vi "CSM Data Type.vi"() -> ()   [LabVIEW 2017]
uses:
  <vilib>/Utility/Data Type/Type Definitions/Data Type.ctl
  user.lib/_NEVSTOP/Communicable State Machine(CSM)/Utility/_support/CSM Data Type String to Enum(String).vi
  user.lib/_NEVSTOP/Communicable State Machine(CSM)/Communicable State Machine.lvlib
  <vilib>/Utility/Data Type/NI_Data Type.lvlib
panel:
  out "Array Dim 12":i32
  out "Secondary Type String 12":string
  out "Primary Type 12":T1
  out "Data Type String 12":string
  out "Array Dim 11":i32
  out "Secondary Type String 11":string
  out "Primary Type 11":T1
  out "Data Type String 11":string
  out "Array Dim 10":i32
  out "Secondary Type String 10":string
  out "Primary Type 10":T1
  out "Data Type String 10":string
  out "Array Dim 9":i32
  out "Secondary Type String 9":string
  out "Primary Type 9":T1
  out "Data Type String 9":string
  out "Array Dim 8":i32
  out "Secondary Type String 8":string
  out "Primary Type 8":T1
  out "Data Type String 8":string
  out "Array Dim 7":i32
  out "Secondary Type String 7":string
  out "Primary Type 7":T1
  out "Data Type String 7":string
  out "Array Dim 6":i32
  out "Secondary Type String 6":string
  out "Primary Type 6":T1
  out "Data Type String 6":string
  out "Array Dim 5":i32
  out "Secondary Type String 5":string
  out "Primary Type 5":T1
  out "Data Type String 5":string
  out "Array Dim 4":i32
  out "Secondary Type String 4":string
  out "Primary Type 4":T1
  out "Data Type String 4":string
  out "Array Dim 3":i32
  out "Secondary Type String 3":string
  out "Primary Type 3":T1
  out "Data Type String 3":string
  out "Array Dim 2":i32
  out "Secondary Type String 2":string
  out "Primary Type 2":T1
  out "Data Type String 2":string
  out "Data Type String":string
  out "Primary Type":T1
  out "Secondary Type String":string
  out "Array Dim":i32
  in  "Data 12":dbl[][](array[numeric])=[[3.12, 4.113, 2.3, 5.0, 5.0, 2.3, 4.11, 5.0]]
  in  "Data 11":T2(array[cluster])=[{"Name"="", "Child"={"Name"="ddd"}, "Bool"=FALSE}, {"Name"="ddd", "Child"={"Name"=""}, "Bool"=TRUE}]
  in  "Data 2":path=path "C:/ni-rt/data/a/2023.07.25"
  in  "Data 10":T3={"Name"="abc", "Child"={"Name"="ddd"}, "Bool"=FALSE}
  in  "Data 9":dbl[](array[numeric])=[3.12, 4.11, 5.0]
  in  "Data 8":enum16{"1 - aaaa", "2 - bbbb", "555 - ccccc"}(ring)=enum."555 - ccccc"
  in  "Data 7":enum16{"1 - aaaa", "2 - bbbb", "555 - ccccc"}(ring)=enum."555 - ccccc"
  in  "Data 6":enum16{"aaaa", "bbbb", "ccccc"}(ring)=enum."bbbb"
  in  "Data 5":dbl=3.1415926
  in  "Data 4":i32=66
  in  "Data 3":bool=TRUE
  in  "Data 1":string="abcd"
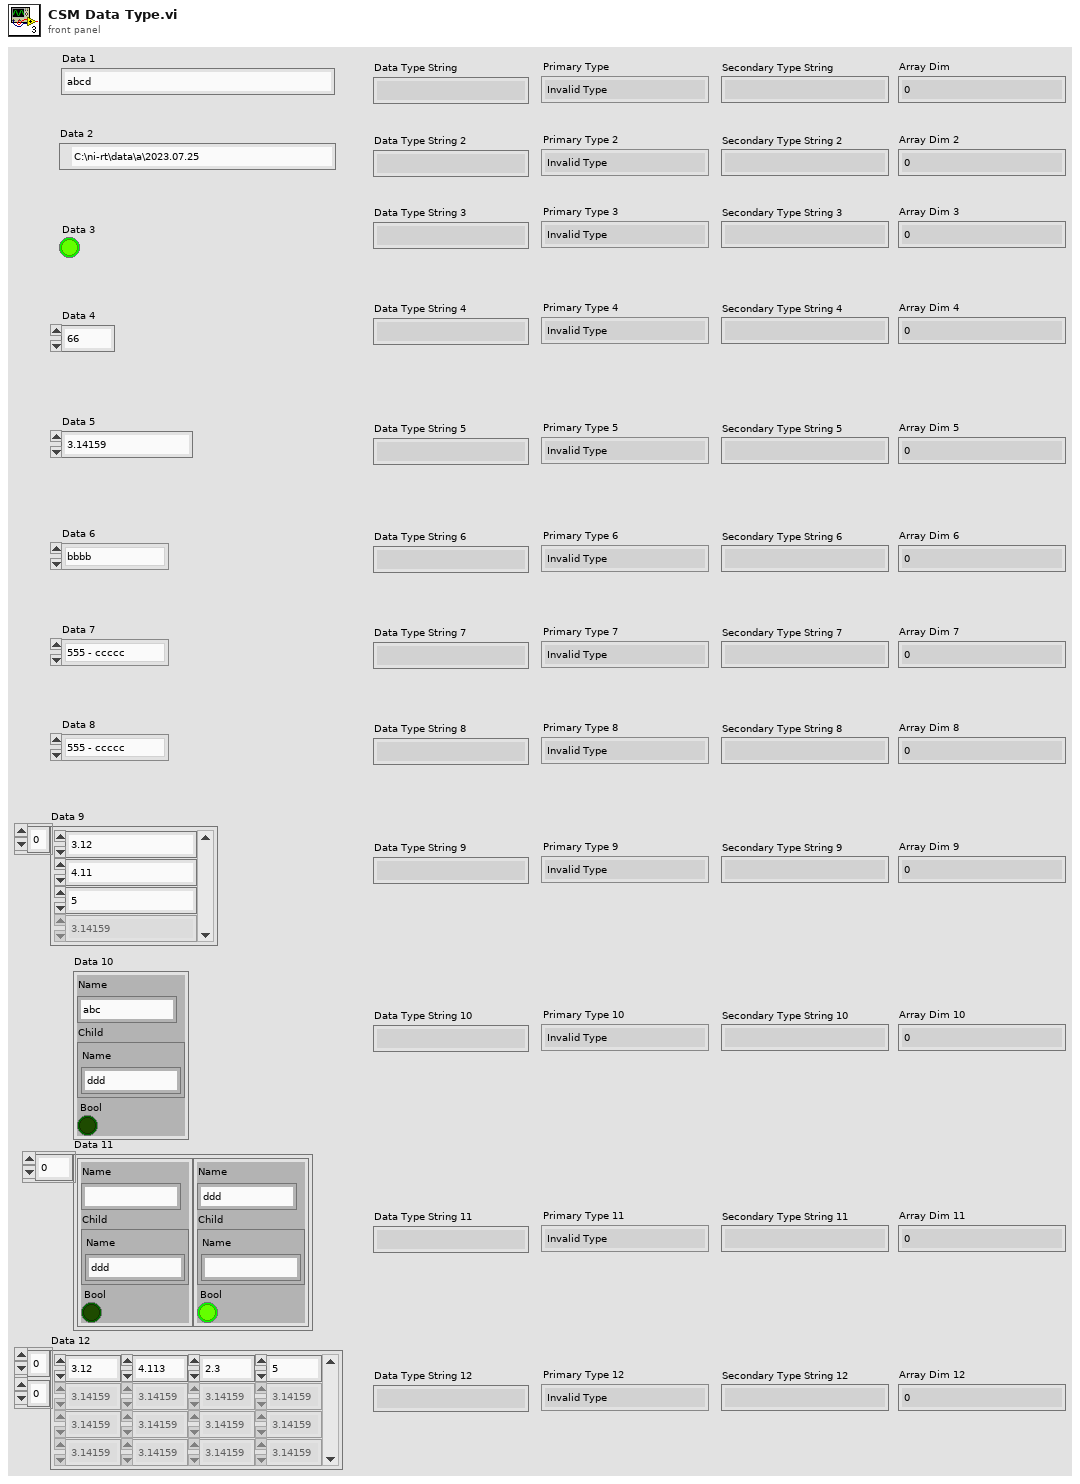
[diagram p1: front panel]
types:
  T1 = typedef "NI_Data Type.lvlib/Data Type.ctl" = enum8{"Invalid Type", "Void", "I8", "I16", "I32", "I64", "U8", "U16", "U32", "U64", "Single Float", "Double Float", "Extended Float", "Single Complex", "Double Complex", "Extended Complex", "Enum U8", "Enum U16", "Enum U32", "Enum U64", "Single Float With Unit", "Double Float With Unit", "Extended Float With Unit", "Single Complex with Unit", "Double Complex with Unit", "Extended Complex with Unit", "Boolean", "String", "Path", "Picture", "Tag", "Array", "Cluster", "Variant", "LV Variant", "Waveform", "Timestamp", "Digital Waveform", "Digital Data", "ExpressData", "Refnum", "External Data", "VI", "Poly VI", "LabVIEW Class Instance", "Fixed Point"}
  T2 = cluster{"Name":string, "Child":cluster{"Name":string}, "Bool":bool}[]
  T3 = cluster{"Name":string, "Child":cluster{"Name":string}, "Bool":bool}
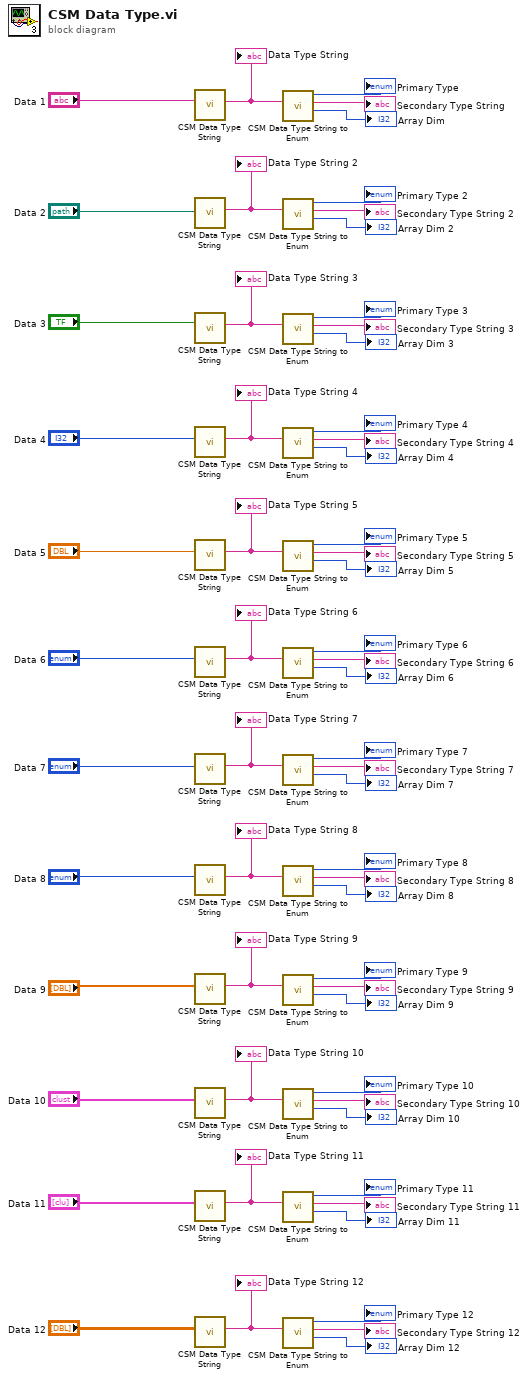
[diagram p0: block diagram]
diagram:
  n1 = call "CSM Data Type String.vi"("Data"="Data 1") -> ("Data Type String"=w60:string)  [unwired: 10 in]
  "Data Type String" <- w60
  n2 = call "CSM Data Type String.vi"("Data"="Data 2") -> ("Data Type String"=w52:string)  [unwired: 10 in]
  "Data Type String 2" <- w52
  n3 = call "CSM Data Type String.vi"("Data"="Data 3") -> ("Data Type String"=w50:string)  [unwired: 10 in]
  "Data Type String 3" <- w50
  n4 = call "CSM Data Type String.vi"("Data"="Data 4") -> ("Data Type String"=w42:string)  [unwired: 10 in]
  "Data Type String 4" <- w42
  n5 = call "CSM Data Type String.vi"("Data"="Data 5") -> ("Data Type String"=w40:string)  [unwired: 10 in]
  "Data Type String 5" <- w40
  n6 = call "CSM Data Type String.vi"("Data"="Data 6") -> ("Data Type String"=w32:string)  [unwired: 10 in]
  "Data Type String 6" <- w32
  n7 = call "CSM Data Type String.vi"("Data"="Data 7") -> ("Data Type String"=w30:string)  [unwired: 10 in]
  "Data Type String 7" <- w30
  n8 = call "CSM Data Type String.vi"("Data"="Data 8") -> ("Data Type String"=w22:string)  [unwired: 10 in]
  "Data Type String 8" <- w22
  n9 = call "CSM Data Type String.vi"("Data"="Data 9") -> ("Data Type String"=w20:string)  [unwired: 10 in]
  "Data Type String 9" <- w20
  n10 = call "CSM Data Type String.vi"("Data"="Data 10") -> ("Data Type String"=w12:string)  [unwired: 10 in]
  "Data Type String 10" <- w12
  n11 = call "CSM Data Type String.vi"("Data"="Data 11") -> ("Data Type String"=w10:string)  [unwired: 10 in]
  "Data Type String 11" <- w10
  n12 = call "CSM Data Type String.vi"("Data"="Data 12") -> ("Data Type String"=w2:string)  [unwired: 10 in]
  "Data Type String 12" <- w2
  n13 = call-poly "CSM Data Type String to Enum.vi"("Data Type String"=w60) -> ("Array Dim"=→"Array Dim":i32, "Secondary Type String"=→"Secondary Type String":string, "Primary Type"=→"Primary Type":T1)  [unwired: 8 in]
  n14 = call-poly "CSM Data Type String to Enum.vi"("Data Type String"=w52) -> ("Array Dim"=→"Array Dim 2":i32, "Secondary Type String"=→"Secondary Type String 2":string, "Primary Type"=→"Primary Type 2":T1)  [unwired: 8 in]
  n15 = call-poly "CSM Data Type String to Enum.vi"("Data Type String"=w50) -> ("Array Dim"=→"Array Dim 3":i32, "Secondary Type String"=→"Secondary Type String 3":string, "Primary Type"=→"Primary Type 3":T1)  [unwired: 8 in]
  n16 = call-poly "CSM Data Type String to Enum.vi"("Data Type String"=w42) -> ("Array Dim"=→"Array Dim 4":i32, "Secondary Type String"=→"Secondary Type String 4":string, "Primary Type"=→"Primary Type 4":T1)  [unwired: 8 in]
  n17 = call-poly "CSM Data Type String to Enum.vi"("Data Type String"=w40) -> ("Array Dim"=→"Array Dim 5":i32, "Secondary Type String"=→"Secondary Type String 5":string, "Primary Type"=→"Primary Type 5":T1)  [unwired: 8 in]
  n18 = call-poly "CSM Data Type String to Enum.vi"("Data Type String"=w32) -> ("Array Dim"=→"Array Dim 6":i32, "Secondary Type String"=→"Secondary Type String 6":string, "Primary Type"=→"Primary Type 6":T1)  [unwired: 8 in]
  n19 = call-poly "CSM Data Type String to Enum.vi"("Data Type String"=w30) -> ("Array Dim"=→"Array Dim 7":i32, "Secondary Type String"=→"Secondary Type String 7":string, "Primary Type"=→"Primary Type 7":T1)  [unwired: 8 in]
  n20 = call-poly "CSM Data Type String to Enum.vi"("Data Type String"=w22) -> ("Array Dim"=→"Array Dim 8":i32, "Secondary Type String"=→"Secondary Type String 8":string, "Primary Type"=→"Primary Type 8":T1)  [unwired: 8 in]
  n21 = call-poly "CSM Data Type String to Enum.vi"("Data Type String"=w20) -> ("Array Dim"=→"Array Dim 9":i32, "Secondary Type String"=→"Secondary Type String 9":string, "Primary Type"=→"Primary Type 9":T1)  [unwired: 8 in]
  n22 = call-poly "CSM Data Type String to Enum.vi"("Data Type String"=w12) -> ("Array Dim"=→"Array Dim 10":i32, "Secondary Type String"=→"Secondary Type String 10":string, "Primary Type"=→"Primary Type 10":T1)  [unwired: 8 in]
  n23 = call-poly "CSM Data Type String to Enum.vi"("Data Type String"=w10) -> ("Array Dim"=→"Array Dim 11":i32, "Secondary Type String"=→"Secondary Type String 11":string, "Primary Type"=→"Primary Type 11":T1)  [unwired: 8 in]
  n24 = call-poly "CSM Data Type String to Enum.vi"("Data Type String"=w2) -> ("Array Dim"=→"Array Dim 12":i32, "Secondary Type String"=→"Secondary Type String 12":string, "Primary Type"=→"Primary Type 12":T1)  [unwired: 8 in]
